vi "Async.Engine.Initialize.vi"(6 "Timeout (ms) (5000)":u16=5000, 7 "Error Log Settings":T1, 8 "error in (no error)":errorcluster, 10 "Processes":cluster{"VI":refnum<vi>, "Parameters":variant}[](array[cluster]), 11 "Custom Device Ref":T2 format="%.0x") -> (0 "error out":errorcluster, 3 "Async":refnum<class "VS Inline Async API.lvclass">)   [LabVIEW 2023, in "VS Inline Async API.lvlib" / "VS Inline Async API.lvclass"]
uses:
  VS Inline Async API.lvclass
  VS Inline Async API.lvclass/VS Inline Async API.ctl
  VS Inline Async API.lvlib
  _Data Access Engine/Data Access Engine/Data Access Engine.lvclass
  <vilib>/NI VeriStand/Custom Device API/Custom Device API.lvlib
  <vilib>/NI VeriStand/Custom Device API/Custom Device Item Ref.ctl
  Types/Error Handling Settings.ctl
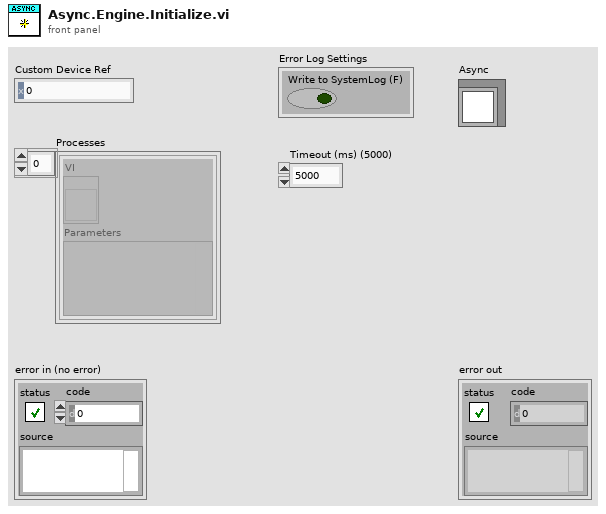
[diagram p1: front panel]
types:
  T1 = typedef "VS Inline Async API.lvlib/VS Inline Async API.lvclass/Error Handling Settings.ctl" = cluster{"Write to SystemLog (F)":bool}
  T2 = typedef "Custom Device API.lvlib/Custom Device Item Ref.ctl" = u64
  T3 = typedef "Custom Device API.lvlib/Custom Device Item Info.ctl" = cluster{"Name":string, "Is Channel":bool, "GUID":string, "Is Waveform":bool}
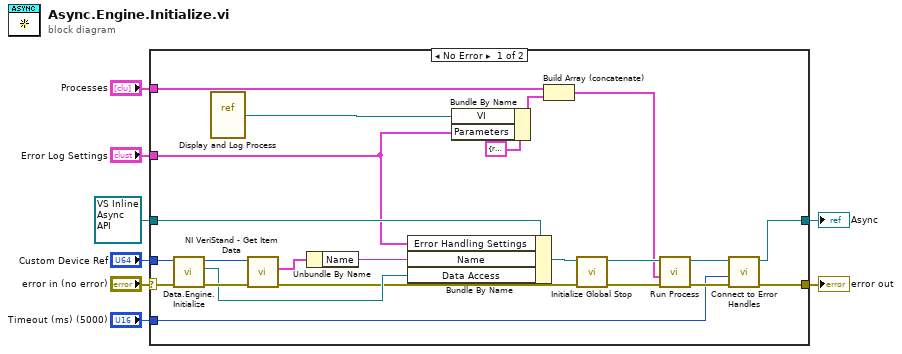
[diagram p0: block diagram]
diagram:
  n1 = case shown="No Error" "error in (no error)" {
    selector: "error in (no error)" -> [w19 w33]
    tunnel: [w28 w33] -> w7
    tunnel: [w26 w32] -> w5
    tunnel: refnum<class "VS Inline Async API.lvclass"> refnum ("Async in") -> [w31 w32]
    tunnel: "Processes" -> [w30 _]
    tunnel: "Custom Device Ref" -> [w18 _]
    tunnel: "Error Log Settings" -> [w10 _]
    tunnel: "Timeout (ms) (5000)" -> [w9 _]
    frame No Error {
      n2 = call "Data.Engine.Initialize.vi"("error in"=w19, "Custom Device Ref"=w18) -> ("error out"=w17:errorcluster, "Data Access Engine"=w13:refnum<class "Data Access Engine.lvclass">, "Custom Device Ref"=w16:T2)  [unwired: 7 in]
      n3 = vi-ref "Display and Log Process.vi"() -> (w24:refnum<vi>)
      n4 = call <vilib>:"NI VeriStand - Get Item Data.vi"("error in (no error)"=w17, "Item Ref in"=w16) -> ("error out"=w12:errorcluster, "Item Info"=w15:T3)  [unwired: 6 in, 2 out]
      n5 = Unbundle By Name(w15) -> ("Name"=w14:string)
      n6 = Bundle By Name(cluster=w31, "Error Handling Settings"=w10, "Name"=w14, "Data Access"=w13) -> (w11:refnum<class "VS Inline Async API.lvclass">)
      n7 = Bundle By Name(cluster=cluster{"VI":refnum<vi>, "Parameters":variant} {"VI"=refnum, "Parameters"=variant} ("Process"), "VI"=w24, "Parameters"=w10) -> (w23:cluster{"VI":refnum<vi>, "Parameters":variant})
      n8 = Build Array (concatenate)(w30, w23) -> (w20:cluster{"VI":refnum<vi>, "Parameters":variant}[])
      n9 = call "Initialize Global Stop.vi"("error in (no error)"=w12, "Async in"=w11) -> ("error out"=w22:errorcluster, "Async out"=w21:refnum<class "VS Inline Async API.lvclass">)  [unwired: 8 in]
      n10 = call "Run Process.vi"("error in (no error)"=w22, "Processes"=w20, "Async in"=w21) -> ("error out"=w29:errorcluster, "Async out"=w27:refnum<class "VS Inline Async API.lvclass">)  [unwired: 7 in]
      n11 = call "Connect to Error Handles.vi"("error in"=w29, "Timeout (ms)"=w9, "Async in"=w27) -> ("error out"=w28:errorcluster, "Async out"=w26:refnum<class "VS Inline Async API.lvclass">)  [unwired: 7 in]
    }
    frame Error {
    }
  }
  "error out" <- w7
  "Async" <- w5
